vi "Error Generator.vi"(8 "error in":errorcluster, 10 "data return (error code)":u8, 11 "function return":T1 items=["Read Discrete Inputs"=2, "Read Coils"=1, "Write Single Coil"=5, "Write Multiple Coils"=15, "Read Input Register"=4, "Read Holding Registers"=3, "Write Single Register"=6, "Write Multiple Registers"=16, "Read/Write Multiple Registers"=23, "Mask Write Register"=22, "Read FIFO Queue"=24, "Read File Record"=20, "Write File Record"=21, "Read Exception Status"=7, "Diagnostic"=8, "Get Com Event Counter"=11, "Get Com Event Log"=12, "Report Slave ID"=17, "Read Device Identification"=43]) -> (0 "error out":errorcluster)   [LabVIEW 2015, in "Modbus Library.lvlib" / "Master Function Definition.lvclass"]
doc: "This VI takes a function error code (>0x80) and its data return and generates a labview error code. The error returned is 900150+Modbus error code."
uses:
  Master Function Definition/Master Function Definition.lvclass
  Modbus Data Unit/Function.ctl
  Modbus Library.lvlib
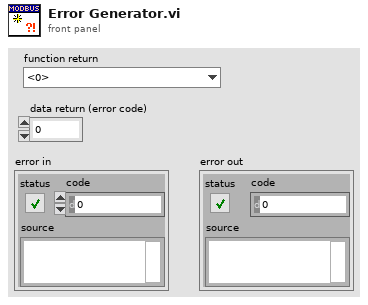
[diagram p1: front panel]
types:
  T1 = typedef "Modbus Library.lvlib/Function.ctl" = u8
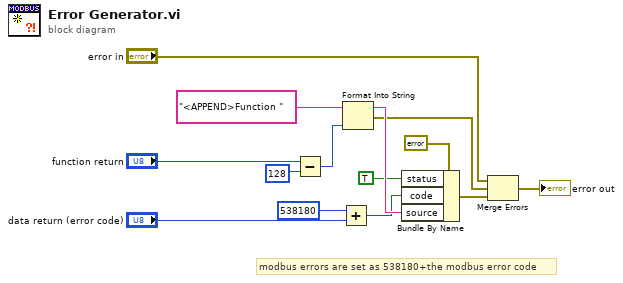
[diagram p0: block diagram]
diagram:
  # "modbus errors are set as 538180+the modbus error code"
  n1 = Subtract(x="function return", y=u8 128) -> (x-y=w14:T1)
  n2 = Add(x=538180, y="data return (error code)") -> (x+y=w8:i32)
  n3 = Format Into String(initial string="<APPEND>Function " ("format string"), w14) -> (resulting string=w10:string, error out=w9:errorcluster)  [unwired: 2 in]
  n4 = Bundle By Name(cluster=errorcluster {"status"=FALSE, "code"=0, "source"=""} ("error constant"), "status"=TRUE, "code"=w8, "source"=w10) -> (w4:errorcluster)
  n5 = Merge Errors("error in", w9, w4) -> (→"error out":errorcluster)
